vi "New.vi"(9 "aggregation method (any)":T2, 10 "match behavior (keep)":T1, 11 "sub-filters":refnum<class "Filter.lvclass">[](array[class])) -> (3 "aggregate filter":refnum<class "Combination.lvclass">)   [LabVIEW 2018, in "Logging.lvlib" / "Combination.lvclass"]
uses:
  Combination.lvclass
  Filter/Filter.lvclass
  C:/Users/Colin/Documents/software_projects/glog/Logging/Filters/Filter/Filter.lvclass
  Aggregation Method.ctl
  Match Behavior.ctl
  Combination.lvclass/Combination.ctl
  Filter/Filter.lvclass/Filter.ctl
  Logging.lvlib
panel:
  # "Connector Pane"
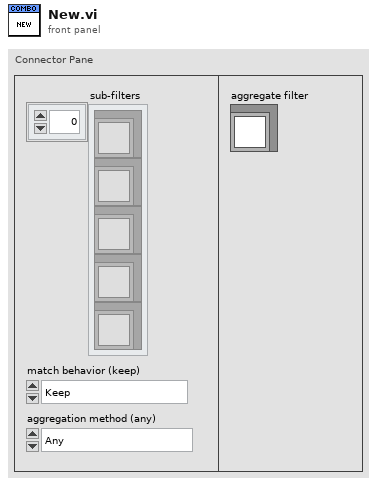
[diagram p1: front panel]
types:
  T1 = typedef "Logging.lvlib/Match Behavior.ctl" = enum16{"Keep", "Discard"}
  T2 = typedef "Logging.lvlib/Aggregation Method.ctl" = enum16{"Any", "Only", "All", "None"}
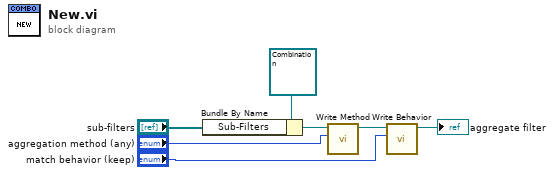
[diagram p0: block diagram]
diagram:
  n1 = Bundle By Name(cluster=refnum<class "Combination.lvclass"> refnum ("Logging.lvlib:And.lvclass"), "Sub-Filters"="sub-filters") -> (w5:refnum<class "Combination.lvclass">)
  n2 = call "Write Method.vi"("Method"="aggregation method (any)", "Filter in"=w5) -> ("Filter out"=w4:refnum<class "Combination.lvclass">)  [unwired: 9 in]
  n3 = call "Write Behavior.vi"("match behavior"="match behavior (keep)", "Filter in"=w4) -> ("Filter out"=→"aggregate filter":refnum<class "Combination.lvclass">)  [unwired: 9 in]
